vi "Routing Channel Page.vi"(8 "error in (no error)":errorcluster, 11 "Node Ptr":T5 format="%.0x") -> (0 "error out":errorcluster)   [LabVIEW 2017, in "Routing and Faulting System Explorer.lvlib"]
uses:
  Routing and Faulting System Explorer.lvlib
  <vilib>/NI Veristand/Custom Device API/Custom Device Item Ref.ctl
  State Control.ctl
  State-Value Row.ctl
  Connection Row.ctl
  Routing Channel Page Controls.ctl
  <vilib>/NI VeriStand/Custom Device API/Custom Device API.lvlib
  Scripting/Routing and Faulting Scripting.lvlib
  Shared/UI Common/UI Common.lvlib
panel:
  in  "Configuration Tab":T1(tab)
  out "State Value":string
  in  "State Name":T2
  out "Connections":T3[](array[typedef])
  out "States":T4[](array[typedef])
  out "Initial State":T2
  out "Routing Channel Name":string
  in  "SHDocVw.IWebBrowser":refnum<k7>(container)
  out "Description":string
  # "Source"
  # "Destination"
  # "State"
  # "State Value"
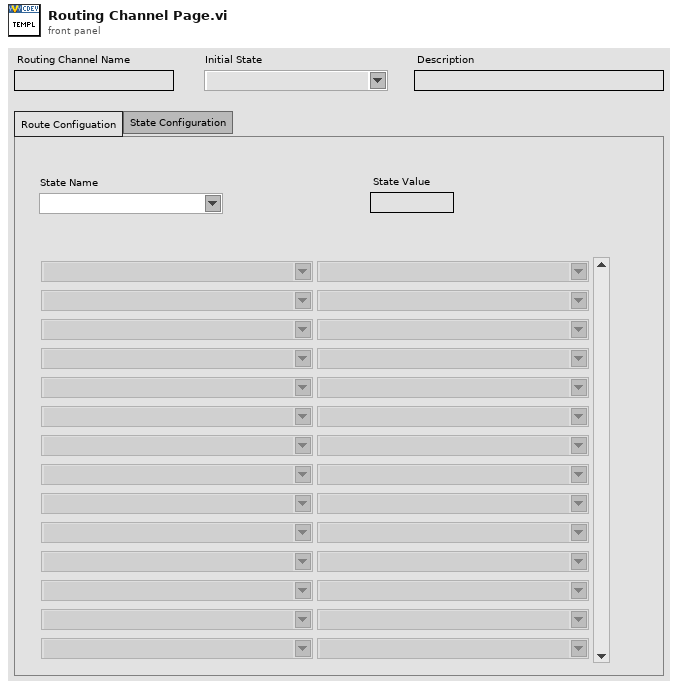
[diagram p1: front panel]
types:
  T1 = enum32{"Route Configuation", "State Configuration"}
  T2 = typedef "Routing and Faulting System Explorer.lvlib/State Control.ctl" = string
  T3 = typedef "Routing and Faulting System Explorer.lvlib/Connection Row.ctl" = cluster{"Source":string, "Destination":string}
  T4 = typedef "Routing and Faulting System Explorer.lvlib/State-Value Row.ctl" = cluster{"State":T2, "State Value":string}
  T5 = typedef "Custom Device API.lvlib/Custom Device Item Ref.ctl" = u64
  T6 = typedef "Routing and Faulting System Explorer.lvlib/Routing Channel Page Controls.ctl" = cluster{"Description":refnum<vi>, "Routing Channel Name":refnum<vi>, "Initial State":refnum<vi>, "Configuration Tab":refnum<vi>, "States":refnum<vi>, "State Value":refnum<vi>, "State Name":refnum<vi>, "Connections":refnum<vi>}
  T7 = typedef "Custom Device API.lvlib/Custom Device Commands.ctl" = enum16{"Default", "Item renamed", "Shutdown", "Dynamic button pressed"}
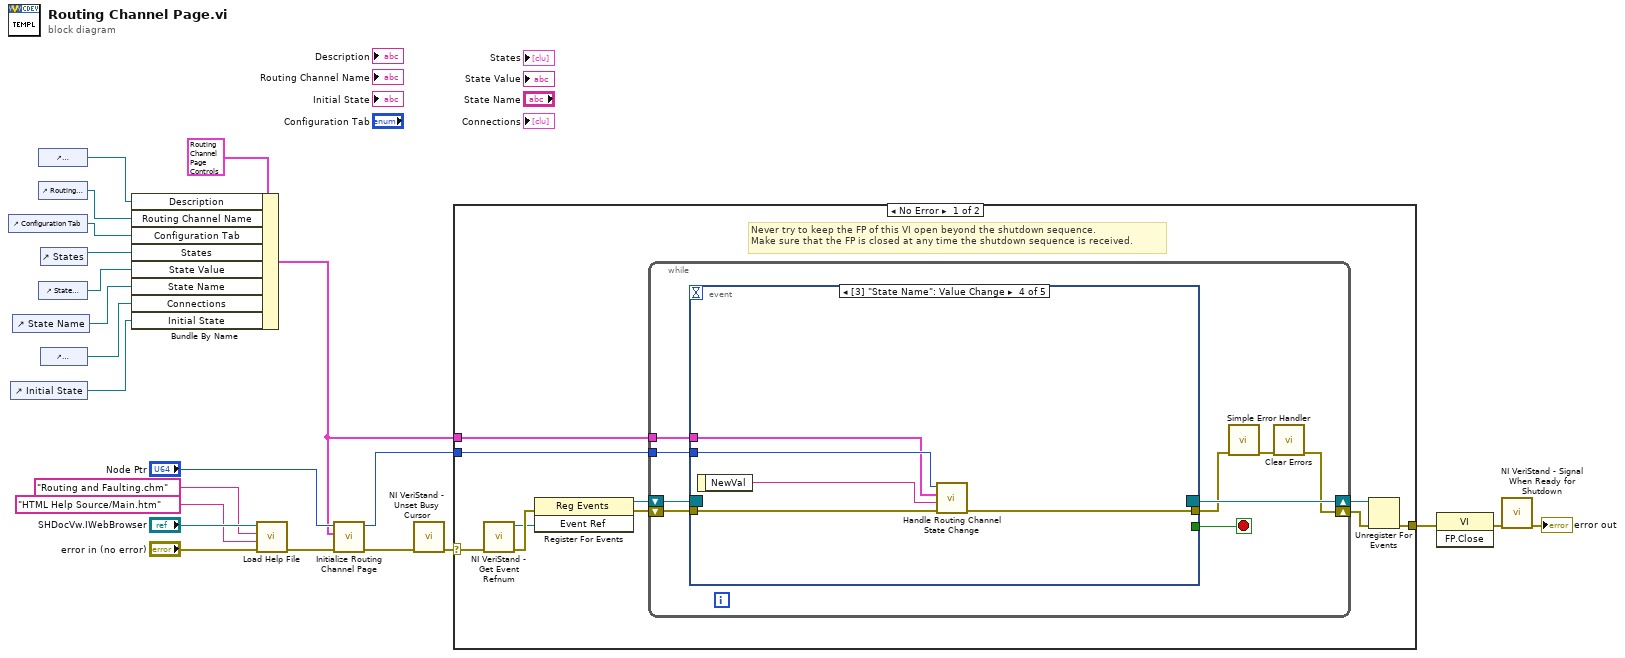
[diagram p0: block diagram]
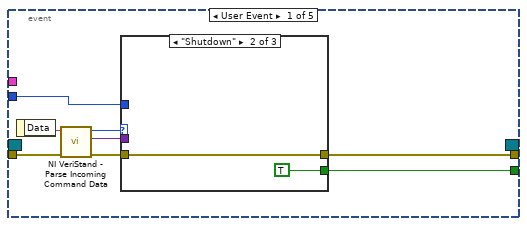
[diagram p2: hidden frame]
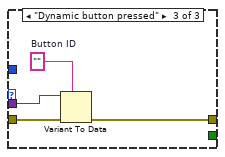
[diagram p4: hidden frame]
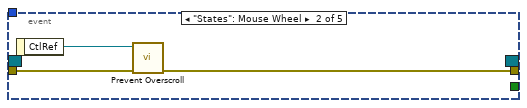
[diagram p5: hidden frame]
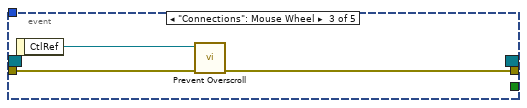
[diagram p6: hidden frame]
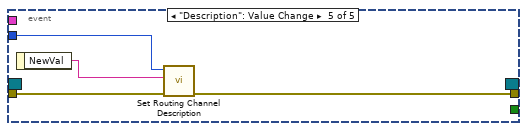
[diagram p7: hidden frame]
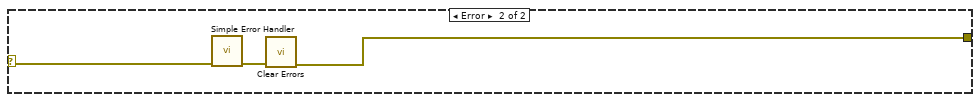
[diagram p8: hidden frame]
diagram:
  n1 = control-ref of="Configuration Tab"() -> (w14:refnum<vi>)
  n2 = control-ref of="Initial State"() -> (w2:refnum<vi>)
  n3 = control-ref of="State Name"() -> (w3:refnum<vi>)
  n4 = control-ref of="Description"() -> (w16:refnum<vi>)
  n5 = control-ref of="Routing Channel Name"() -> (w15:refnum<vi>)
  n6 = control-ref of="State Value"() -> (w12:refnum<vi>)
  n7 = control-ref of="States"() -> (w13:refnum<vi>)
  n8 = control-ref of="Connections"() -> (w4:refnum<vi>)
  n9 = Bundle By Name(cluster=T6 {"Description"=refnum, "Routing Channel Name"=refnum, "Initial State"=refnum, "Configuration Tab"=refnum, "States"=refnum, "State Value"=refnum, "State Name"=refnum, "Connections"=refnum} ("Routing Channel Page Controls"), "Description"=w16, "Routing Channel Name"=w15, "Configuration Tab"=w14, "States"=w13, "State Value"=w12, "State Name"=w3, "Connections"=w4, "Initial State"=w2) -> (w1:T6)
  n10 = call "Load Help File.vi"("error in (no error)"="error in (no error)", "HTML File to Load"="HTML Help Source/Main.htm" ("HTML File"), "Main CHM File"="Routing and Faulting.chm" ("CD_CHM_FileName"), "Browser"="SHDocVw.IWebBrowser") -> ("error out"=w6:errorcluster)  [unwired: 7 in]
  n11 = call "Initialize Routing Channel Page.vi"("error in (no error)"=w6, "Routing Channel Page Controls"=w1, "Routing Channel Ref in"="Node Ptr") -> ("error out"=w22:errorcluster, "Routing Channel Ref out"=w21:T5)  [unwired: 7 in]
  n12 = call <vilib>:"NI VeriStand - Unset Busy Cursor.vi"("error in (no error)"=w22) -> ("error out"=w17:errorcluster)  [unwired: 10 out]
  n13 = case shown="No Error" w17 {
    selector: w17 -> [w24 w74]
    tunnel: [w29 w72] -> w20
    tunnel: w21 -> [w25 _]
    tunnel: w1 -> [w23 _]
    frame No Error {
      # "Never try to keep the FP of this VI open beyond the shutdown sequence.\nMake sure that the FP is closed at any time the shutdown sequence is received."
      n14 = call <vilib>:"NI VeriStand - Get Event Refnum.vi"("error in (no error)"=w24) -> ("error out"=w32:errorcluster, "Event Ref"=w28:refnum<user-event>)  [unwired: 9 out]
      n15 = register-events(error in=w32, w28) -> (reference out=w26:refnum<event-registration>, error out=w27:errorcluster)  [unwired: 1 in]
      n16 = while {
        tunnel: w25 -> [w37]
        shift-right: [w34] -> w30
        shift-left: w27 -> [w40]
        shift-right: [w41] -> w31
        shift-left: w26 -> [w39]
        tunnel: w23 -> [w33]
        stop <- w38 stop-if-true
        n17 = event shown="[3] \"State Name\": Value Change" {
          selector: w39 -> [_ _ _ _ _]
          dyn-events: [_ _ _ _ _] -> w41
          timeout: _ -> [_ _ _ _ _]
          tunnel: w40 -> [w49 w58 w61 w64 w70]
          tunnel: [w45 _ _ _ _] -> w38
          tunnel: [w44 w57 w60 w63 w69] -> w36
          tunnel: w37 -> [w43 _ _ w67 w71]
          tunnel: w33 -> [_ _ _ w65 _]
          event User Event {
            n18 = event-data() -> ("Data"=w48:string)  [unwired: 1 out]
            n19 = call <vilib>:"NI VeriStand - Parse Incoming Command Data.vi"("error in (no error)"=w49, "Incoming data"=w48) -> ("error out"=w47:errorcluster, "Outgoing data"=w42:variant, "Action"=w46:T7)  [unwired: 7 out]
            n20 = case shown="\"Shutdown\"" w46 {
              tunnel: w47 -> [w50 w51 w56]
              tunnel: [_ TRUE _] -> w45
              tunnel: [w50 w51 w53] -> w44
              tunnel: w43 -> [_ _ _]
              tunnel: w42 -> [_ _ w55]
              frame "Default", Default {
              }
              frame "Shutdown" {
              }
              frame "Dynamic button pressed" {
                w54 = ""  # Button ID
                n21 = Variant To Data(error in=w56, type=w54, Variant=w55) -> (error out=w53:errorcluster)  [unwired: 1 out]
              }
            }
          }
          event "States": Mouse Wheel {
            n22 = event-data() -> ("CtlRef"=w59:refnum<vi>)  [unwired: 1 out]
            n23 = call "Prevent Overscroll.vi"("error in (no error)"=w58, "Array Refnum"=w59) -> ("error out"=w57:errorcluster)  [unwired: 8 in, 1 out]
          }
          event "Connections": Mouse Wheel {
            n24 = event-data() -> ("CtlRef"=w62:refnum<vi>)  [unwired: 1 out]
            n25 = call "Prevent Overscroll.vi"("error in (no error)"=w61, "Array Refnum"=w62) -> ("error out"=w60:errorcluster)  [unwired: 8 in, 1 out]
          }
          event Value Change {
            n26 = event-data() -> ("NewVal"=w66:T2)  [unwired: 1 out]
            n27 = call "Handle Routing Channel State Change.vi"("error in (no error)"=w64, "State"=w66, "Routing Channel Page Controls"=w65, "Routing Channel Ref in"=w67) -> ("error out"=w63:errorcluster)  [unwired: 6 in, 1 out]
          }
          event "Description": Value Change {
            n28 = event-data() -> ("NewVal"=w68:string)  [unwired: 1 out]
            n29 = call "Set Routing Channel Description.vi"("error in (no error)"=w70, "New Description"=w68, "Channel Ref in"=w71) -> ("error out"=w69:errorcluster)  [unwired: 7 in, 1 out]
          }
        }
        n30 = call <vilib>:"Simple Error Handler.vi"("error in (no error)"=w36) -> ("error out"=w35:errorcluster)  [unwired: 1 in, 7 out]
        n31 = call <vilib>:"Clear Errors.vi"("error in (no error)"=w35) -> ("error out"=w34:errorcluster)  [unwired: 1 in, 5 out]
      }
      n32 = Unregister For Events(event registration refnum=w31, error in=w30) -> (error out=w29:errorcluster)
    }
    frame Error {
      n33 = call <vilib>:"Simple Error Handler.vi"("error in (no error)"=w74) -> ("error out"=w73:errorcluster)  [unwired: 1 in, 7 out]
      n34 = call <vilib>:"Clear Errors.vi"("error in (no error)"=w73) -> ("error out"=w72:errorcluster)  [unwired: 1 in, 5 out]
    }
  }
  n35 = invoke class="VI" method="FP.Close"(error in=w20) -> (error out=w19:errorcluster)  [unwired: 2 in, 2 out]
  n36 = call <vilib>:"NI VeriStand - Signal When Ready for Shutdown.vi"("error in (no error)"=w19) -> ("error out"=→"error out":errorcluster)  [unwired: 10 out]
